vi "Add Control to Server ClusterDef.vi"(5 "New Control Label":string, 6 "Clear Previous ?(F)":bool, 7 "Source Control ref in":refnum<vi>, 8 "error in (no error)":errorcluster, 10 "Target ClusterDef Name":string, 11 "Server class in":refnum<vi>) -> (0 "error out":errorcluster, 3 "Server class out":refnum<vi>)   [LabVIEW 2019, in "gRPC Scripting Tools.lvlib"]
uses:
  gRPC Scripting Tools.lvlib
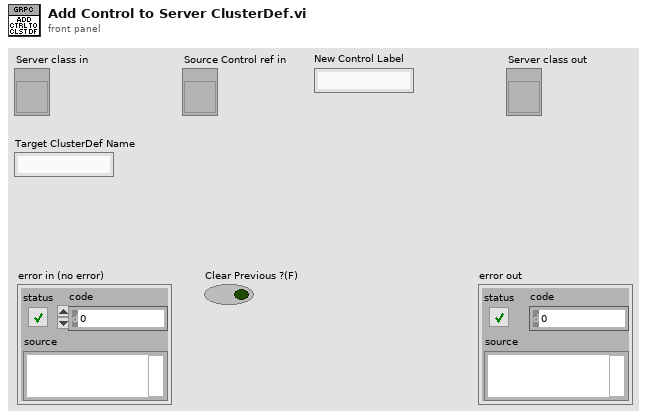
[diagram p1: front panel]
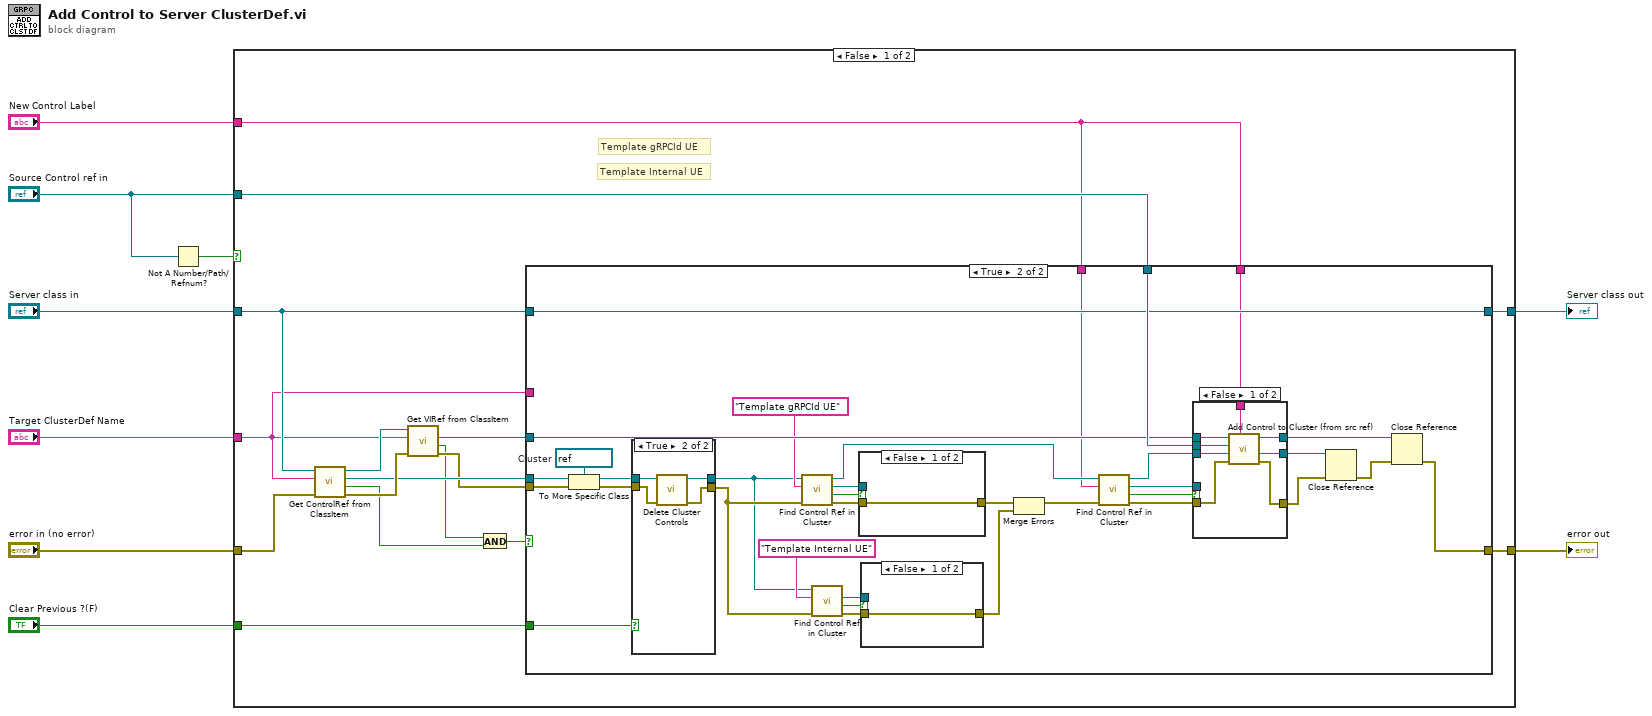
[diagram p0: block diagram]
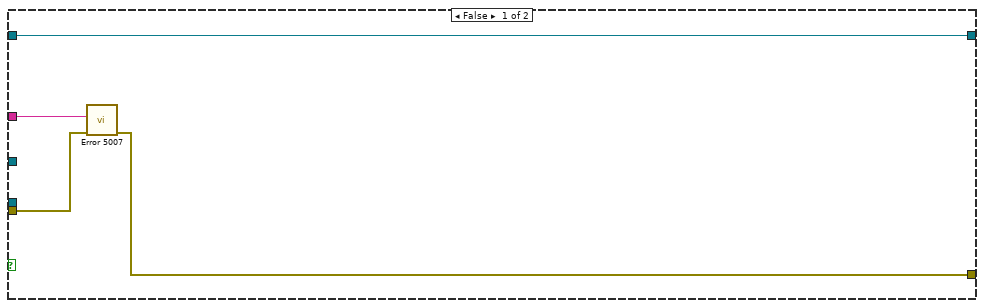
[diagram p2: hidden frame]
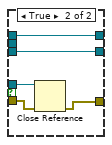
[diagram p3: hidden frame]
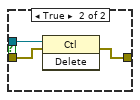
[diagram p4: hidden frame]
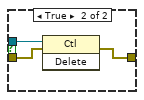
[diagram p5: hidden frame]
diagram:
  n1 = Not A Number/Path/Refnum?(number/path/refnum="Source Control ref in") -> (NaN/Path/Refnum?=w1:bool)
  n2 = case shown="False" w1 {
    tunnel: [w25 w91] -> w9
    tunnel: "Target ClusterDef Name" -> [w10 _]
    tunnel: "error in (no error)" -> [w20 w91]
    tunnel: "New Control Label" -> [w11 _]
    tunnel: "Server class in" -> [w15 w92]
    tunnel: [w14 w92] -> w4
    tunnel: "Clear Previous ?(F)" -> [w13 _]
    tunnel: "Source Control ref in" -> [w12 _]
    frame False {
      # "Template Internal UE"
      # "Template gRPCId UE"
      n3 = call "Get ControlRef from ClassItem.vi"("error in (no error)"=w20, "Item Name"=w10, "LVClassLibrary in"=w15) -> ("error out"=w22:errorcluster, "Found ?"=w18:bool, "Control ref out"=w21:refnum<vi>, "LVClassLibrary out"=w23:refnum<vi>)  [unwired: 5 in]
      n4 = call "Get VIRef from ClassItem.vi"("error in (no error)"=w22, "Item Name"=w10, "LVClassLibrary in"=w23) -> ("error out"=w19:errorcluster, "Found ?"=w17:bool, "VIref out"=w24:refnum<vi>)  [unwired: 5 in, 1 out]
      n5 = And(x=w17, y=w18) -> (x .and. y?=w16:bool)
      n6 = case shown="True" w16 {
        tunnel: [w27 w30] -> w25
        tunnel: w12 -> [_ w63]
        tunnel: w24 -> [_ w62]
        tunnel: w21 -> [_ w61]
        tunnel: w19 -> [w28 w59]
        tunnel: w15 -> [w29 w58]
        tunnel: [w29 w58] -> w14
        tunnel: w13 -> [_ w55]
        tunnel: w11 -> [_ w40]
        tunnel: w11 -> [_ w35]
        tunnel: w10 -> [w26 _]
        frame False {
          n7 = call "Error 5007.vi"("error in (no error)"=w28, "Target ClusterDef Name"=w26) -> ("error out"=w27:errorcluster)  [unwired: 9 in]
        }
        frame True {
          w60 = refnum<vi> refnum  # Cluster
          n8 = To More Specific Class(target class=w60, reference=w61, error in=w59) -> (specific class reference=w57:refnum<vi>, error out=w56:errorcluster)
          n9 = case shown="True" w55 {
            tunnel: w57 -> [w86 w90]
            tunnel: w56 -> [w85 w89]
            tunnel: [w86 w88] -> w45
            tunnel: [w85 w87] -> w46
            frame False {
            }
            frame True {
              n10 = call "Delete Cluster Controls.vi"("error in (no error)"=w89, "Cluster in"=w90) -> ("error out"=w87:errorcluster, "Cluster out"=w88:refnum<vi>)  [unwired: 8 in]
            }
          }
          n11 = call "Find Control Ref in Cluster.vi"("error in (no error)"=w46, "Control Name"="Template gRPCId UE", "Cluster ref in"=w45) -> ("error out"=w51:errorcluster, "Found ?"=w53:bool, "Ctl ref"=w52:refnum<vi>, "Cluster ref out"=w41:refnum<vi>)  [unwired: 5 in]
          n12 = call "Find Control Ref in Cluster.vi"("error in (no error)"=w46, "Control Name"="Template Internal UE", "Cluster ref in"=w45) -> ("error out"=w50:errorcluster, "Found ?"=w48:bool, "Ctl ref"=w49:refnum<vi>)  [unwired: 5 in, 1 out]
          n13 = case shown="False" w53 {
            tunnel: w52 -> [_ w84]
            tunnel: w51 -> [w81 w83]
            tunnel: [w81 w82] -> w44
            frame False {
            }
            frame True {
              n14 = invoke class="Ctl" method="Delete"(reference=w84, error in=w83) -> (error out=w82:errorcluster)  [unwired: 1 in, 2 out]
            }
          }
          n15 = case shown="False" w48 {
            tunnel: w49 -> [_ w80]
            tunnel: w50 -> [w77 w79]
            tunnel: [w77 w78] -> w43
            frame False {
            }
            frame True {
              n16 = invoke class="Ctl" method="Delete"(reference=w80, error in=w79) -> (error out=w78:errorcluster)  [unwired: 1 in, 2 out]
            }
          }
          n17 = Merge Errors(w44, w43) -> (w42:errorcluster)
          n18 = call "Find Control Ref in Cluster.vi"("error in (no error)"=w42, "Control Name"=w40, "Cluster ref in"=w41) -> ("error out"=w38:errorcluster, "Found ?"=w37:bool, "Ctl ref"=w36:refnum<vi>, "Cluster ref out"=w39:refnum<vi>)  [unwired: 5 in]
          n19 = case shown="False" w37 {
            tunnel: [w67 w74] -> w33
            tunnel: w63 -> [w71 _]
            tunnel: w62 -> [w70 w72]
            tunnel: w39 -> [w69 w73]
            tunnel: w38 -> [w68 w75]
            tunnel: w36 -> [_ w76]
            tunnel: w35 -> [w66 _]
            tunnel: [w64 w73] -> w32
            tunnel: [w65 w72] -> w31
            frame False {
              n20 = call "Add Control to Cluster (from src ref).vi"("New Control Label"=w66, "error in (no error)"=w68, "Cluster ref in (owner)"=w69, "Source control ref in"=w71, "Owning VI ref in"=w70) -> ("error out"=w67:errorcluster, "Cluster ref out (owner)"=w64:refnum<vi>, "Owning VI ref out"=w65:refnum<vi>)  [unwired: 3 in, 1 out]
            }
            frame True {
              n21 = Close Reference(reference=w76, error in (no error)=w75) -> (error out=w74:errorcluster)
            }
          }
          n22 = Close Reference(reference=w32, error in (no error)=w33) -> (error out=w34:errorcluster)
          n23 = Close Reference(reference=w31, error in (no error)=w34) -> (error out=w30:errorcluster)
        }
      }
    }
    frame True {
    }
  }
  "error out" <- w9
  "Server class out" <- w4
